vi "Calculate Starting Voltages.vi"(10 "output cluster":T1, 11 "Boolean in":refnum<vi>) -> ()   [LabVIEW 2016]
uses:
  Controls/Cal Refs.ctl
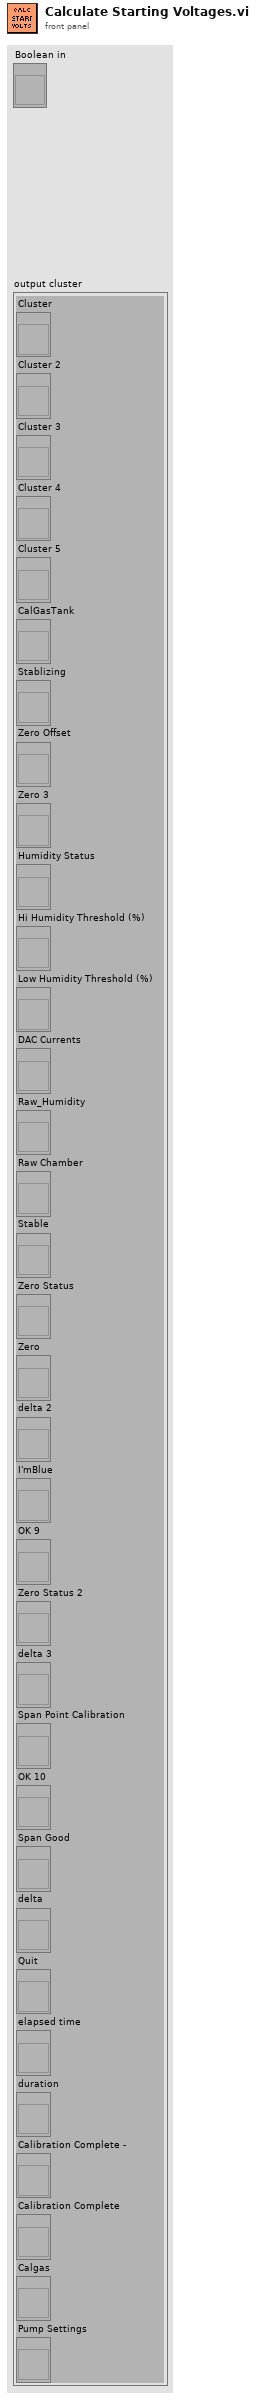
[diagram p1: front panel]
types:
  T1 = typedef "Cal Refs.ctl" = cluster{"Cluster":refnum<vi>, "Cluster 2":refnum<vi>, "Cluster 3":refnum<vi>, "Cluster 4":refnum<vi>, "Cluster 5":refnum<vi>, "CalGasTank":refnum<vi>, "Stablizing":refnum<vi>, "Zero Offset":refnum<vi>, "Zero 3":refnum<vi>, "Humidity Status":refnum<vi>, "Hi Humidity Threshold (%)":refnum<vi>, "Low Humidity Threshold (%)":refnum<vi>, "DAC Currents":refnum<vi>, "Raw_Humidity":refnum<vi>, "Raw Chamber":refnum<vi>, "Stable":refnum<vi>, "Zero Status":refnum<vi>, "Zero":refnum<vi>, "delta 2":refnum<vi>, "I'mBlue":refnum<vi>, "OK 9":refnum<vi>, "Zero Status 2":refnum<vi>, "delta 3":refnum<vi>, "Span Point Calibration":refnum<vi>, "OK 10":refnum<vi>, "Span Good":refnum<vi>, "delta":refnum<vi>, "Quit":refnum<vi>, "elapsed time":refnum<vi>, "duration":refnum<vi>, "Calibration Complete -":refnum<vi>, "Calibration Complete":refnum<vi>, "Calgas":refnum<vi>, "Pump Settings":refnum<vi>}
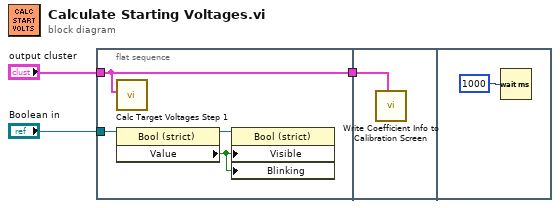
[diagram p0: block diagram]
diagram:
  n1 = flat-sequence {
    tunnel: "output cluster" -> [w6]
    tunnel: [w6] -> w1
    tunnel: "Boolean in" -> [w4]
    tunnel: w1 -> [w8]
    frame #0 {
      n2 = call "Calc Target Voltages Step 1.vi"("output cluster"=w6) -> ()  [unwired: 11 in]
      n3 = property class="Bool (strict)"(reference=w4) -> (reference out=w5:refnum<vi>, "Value"=w7:bool)  [unwired: 1 in, 1 out]
      n4 = property on="Property Node" class="Bool (strict)"(reference=w5, "Visible"=w7, "Blinking"=w7) -> ()  [unwired: 1 in, 2 out]
    }
    frame #1 {
      n5 = call "Write Coefficient Info to Calibration Screen.vi"("output cluster"=w8) -> ()  [unwired: 10 in, 1 out]
    }
    frame #2 {
      n6 = Wait (ms)(milliseconds to wait=u32 1000) -> ()  [unwired: 1 out]
    }
  }
